vi "SelectStageTrajectory.vi"(6 "Stage Position Limit":i32=360, 10 "New Stage Position":i32, 11 "Current Stage Position":dbl) -> (3 "Target Position":dbl)   [LabVIEW 2013]
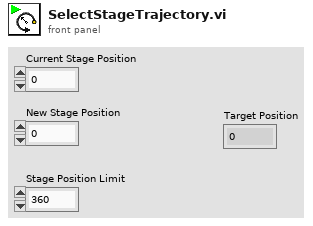
[diagram p1: front panel]
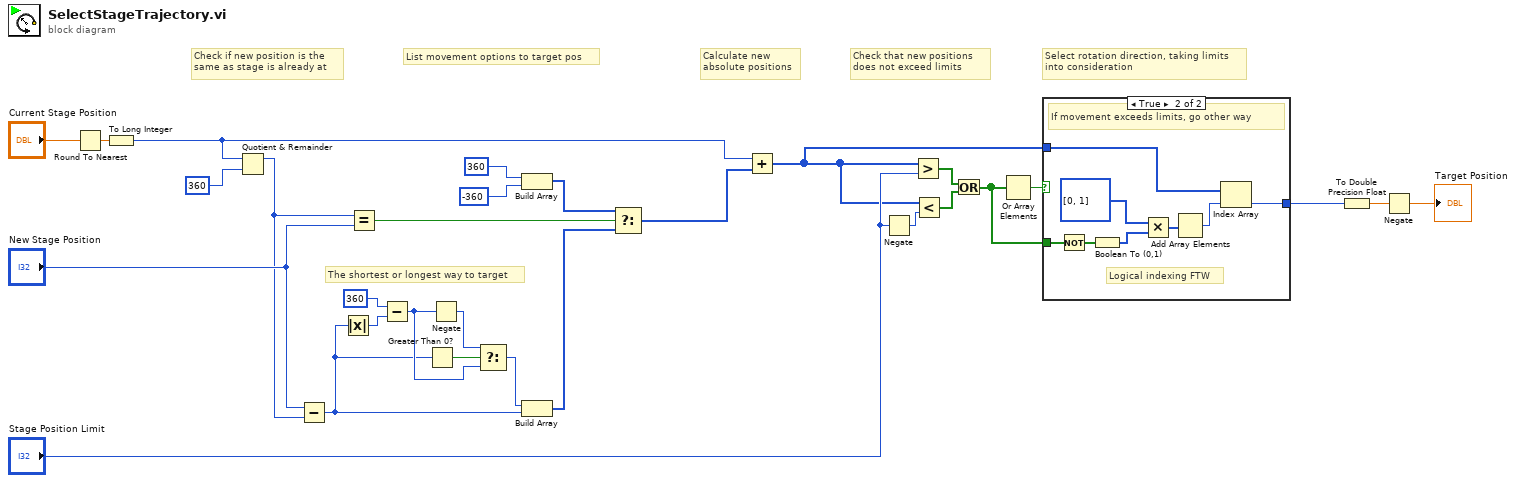
[diagram p0: block diagram]
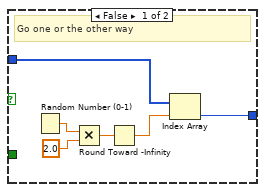
[diagram p2: hidden frame]
diagram:
  # "Calculate new \nabsolute positions"
  # "Select rotation direction, taking limits \ninto consideration"
  # "Check that new positions \ndoes not exceed limits"
  # "The shortest or longest way to target"
  # "List movement options to target pos"
  # "Check if new position is the \nsame as stage is already at"
  n1 = Round To Nearest(number="Current Stage Position") -> (nearest integer value=w28:dbl)
  n2 = To Long Integer(number=w28) -> (32bit integer=w3:i32)
  n3 = Quotient & Remainder(x=w3, y=360) -> (x-y*floor(x/y)=w21:i32)  [unwired: 1 out]
  n4 = Subtract(x="New Stage Position", y=w21) -> (x-y=w12:i32)
  n5 = Absolute Value(x=w12) -> (abs(x)=w18:i32)
  n6 = Equal?(x=w21, y="New Stage Position") -> (x = y?=w26:bool)
  n7 = Subtract(x=360, y=w18) -> (x-y=w16:i32)
  n8 = Greater Than 0?(x=w12) -> (x > 0?=w20:bool)
  n9 = Negate(x=w16) -> (-x=w17:i32)
  n10 = Select(t=w17, s=w20, f=w16) -> (s? t:f=w11:i32)
  n11 = Build Array(360 ("y"), -360 ("f")) -> (w13:i32[])
  n12 = Build Array(w11, w12) -> (w10:i32[])
  n13 = Select(t=w13, s=w26, f=w10) -> (s? t:f=w23:i32[])
  n14 = Add(x=w3, y=w23) -> (x+y=w9:i32[])
  n15 = Negate(x="Stage Position Limit") -> (-x=w24:i32)
  n16 = Greater?(x=w9, y="Stage Position Limit") -> (0:w8:bool[])
  n17 = Less?(x=w9, y=w24) -> (x < y?=w7:bool[])
  n18 = Or(x=w8, y=w7) -> (x .or. y?=w5:bool[])
  n19 = Or Array Elements(Boolean array=w5) -> (logical OR=w6:bool)
  n20 = case shown="True" w6 {
    tunnel: w9 -> [w32 w43]
    tunnel: w5 -> [_ w41]
    tunnel: [w30 w42] -> w4
    frame False {
      # "Go one or the other way"
      n21 = Random Number (0-1)() -> (number: 0 to 1=w35:dbl)
      n22 = Multiply(x=w35, y=2.0) -> (x*y=w33:dbl)
      n23 = Round Toward -Infinity(1:w33) -> (0:w31:dbl)
      n24 = Index Array(array=w32, index=w31) -> (element=w30:i32)
    }
    frame True {
      # "Logical indexing FTW"
      # "If movement exceeds limits, go other way"
      n25 = Not(x=w41) -> (.not. x?=w40:bool[])
      n26 = Boolean To (0,1)(Boolean=w40) -> (0, 1=w38:i16[])
      n27 = Multiply(x=i32[] [0, 1], y=w38) -> (x*y=w37:i32[])
      n28 = Add Array Elements(numeric array=w37) -> (sum=w36:i32)
      n29 = Index Array(array=w43, index=w36) -> (element=w42:i32)
    }
  }
  n30 = To Double Precision Float(number=w4) -> (double precision float=w2:dbl)
  n31 = Negate(x=w2) -> (-x=→"Target Position":dbl)
